vi "Manual Control - Load (SubVI).vi"(10 "Load name":string, 11 "Digital in":refnum<vi>) -> (3 "shared variable refnum out":dbl)   [LabVIEW 2019]
uses:
  Controls/FGV States.ctl
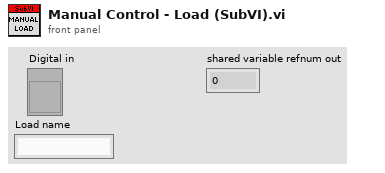
[diagram p1: front panel]
types:
  T1 = typedef "FGV States.ctl" = enum16{"Read", "Write"}
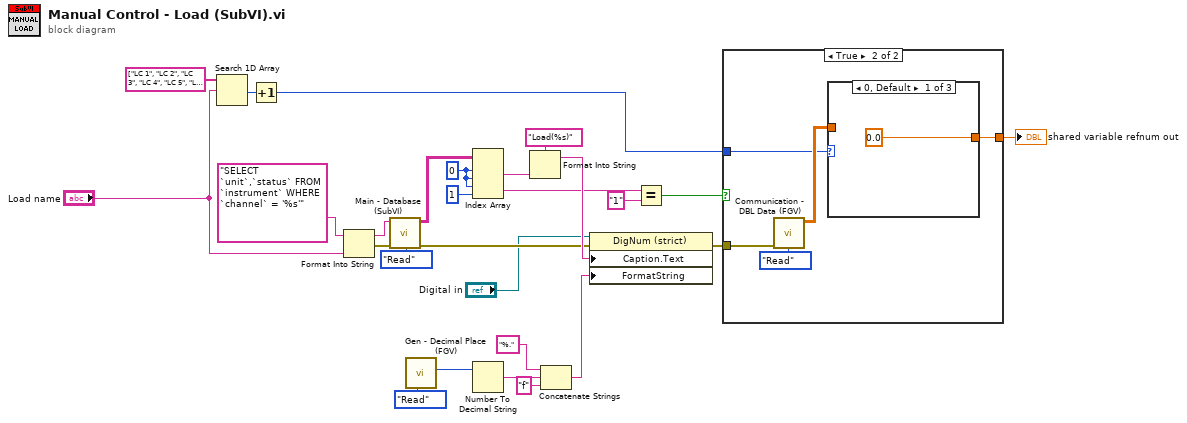
[diagram p0: block diagram]
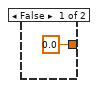
[diagram p2: hidden frame]
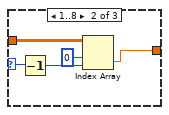
[diagram p3: hidden frame]
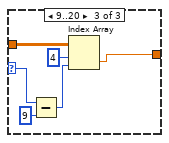
[diagram p4: hidden frame]
diagram:
  w6 = 0 ("index (row)")
  n1 = Search 1D Array(1D array=string[] ["LC 1", "LC 2", "LC 3", "LC 4", "LC 5", "LC 6", "LC 7", "LC 8", "TD 1", "TD 2", "TD 3", "TD 4", "TD 5", "TD 6", "TD 7", "TD 8", "TD 9", "TD 10", "TD 11", "TD 12"], element="Load name") -> (index of element=w15:i32)  [unwired: 1 in]
  n2 = Increment(x=w15) -> (x+1=w14:i32)
  n3 = Format Into String(format string="SELECT `unit`,`status` FROM `instrument` WHERE `channel` = '%s'" ("source"), "Load name") -> (resulting string=w19:string, error out=w18:errorcluster)  [unwired: 2 in]
  n4 = call "Main - Database (SubVI).vi"("Enum"=FGV_States."Read", "error in (no error)"=w18, "SQL query"=w19) -> ("error out"=w23:errorcluster, "data"=w22:string[][])  [unwired: 7 in]
  n5 = call "Gen - Decimal Place (FGV).vi"("Action"=FGV_States."Read") -> ("Ch2 out"=w1:u8)  [unwired: 8 in, 2 out]
  n6 = Index Array(array=w22, index (row) #1=w6, index (col) #1=w6, index (row) #2=w6, index (col) #2=1 ("index (col)")) -> (element #1=w26:string, element #2=w5:string)
  n7 = Number To Decimal String(number=w1) -> (decimal integer string=w12:string)  [unwired: 1 in]
  n8 = Format Into String(format string="Load(%s)" ("initial string"), w26) -> (resulting string=w27:string)  [unwired: 2 in, 1 out]
  n9 = Concatenate Strings("%." ("Format String"), w12, "f" ("string")) -> (w8:string)
  n10 = property on="Property Node" class="DigNum (strict)"(reference="Digital in", error in=w23, "Caption.Text"=w27, "FormatString"=w8) -> (error out=w24:errorcluster)  [unwired: 1 out]
  n11 = Equal?(x=w5, y="1") -> (x = y?=w3:bool)
  n12 = case shown="True" w3 {
    tunnel: w24 -> [_ w33]
    tunnel: [0.0 ("shared variable refnum in") w31] -> w17
    tunnel: w14 -> [_ w29]
    frame False {
    }
    frame True {
      n13 = call "Communication - DBL Data (FGV).vi"("Action"=FGV_States."Read", "error in (no error)"=w33) -> ("DBL SV Out"=w32:dbl[][])  [unwired: 8 in, 1 out]
      n14 = case shown="0, Default" w29 {
        selector: w29 -> [_ w39 w45]
        tunnel: [0.0 ("Numeric") w35 w40] -> w31
        tunnel: w32 -> [_ w38 w43]
        frame 0, Default {
        }
        frame 1..8 {
          n15 = Decrement(x=w39) -> (x-1=w37:i32)
          n16 = Index Array(array=w38, index (row)=0 ("disabled index (row)"), index (col)=w37) -> (element=w35:dbl)
        }
        frame 9..20 {
          n17 = Subtract(x=w45, y=9) -> (x-y=w42:i32)
          n18 = Index Array(array=w43, index (row)=4 ("disabled index (row)"), index (col)=w42) -> (element=w40:dbl)
        }
      }
    }
  }
  "shared variable refnum out" <- w17
